vi "test Float Data Integrity.vi"(8 "error in (no error)":errorcluster, 11 "TestCase in":refnum<class "TestCase.lvclass">) -> (0 "error out":errorcluster, 3 "TestCase out":refnum<class "TestCase.lvclass">)   [LabVIEW 2017, in "Pointer Tests.lvlib" / "Data Manipulation Tests.lvclass"]
uses:
  Data Manipulation Tests.lvclass
  <vilib>/addons/_JKI Toolkits/VI Tester/TestCase.llb/TestCase.lvclass
  Source/Classes/Pointer/Write 1D SGL.vi
  Source/Classes/Pointer/Write 1D DBL.vi
  Source/Classes/Pointer/Write SGL.vi
  Source/Classes/Pointer/Write DBL.vi
  Source/Classes/Pointer/Pointer.lvclass
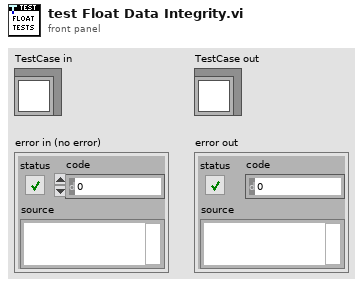
[diagram p1: front panel]
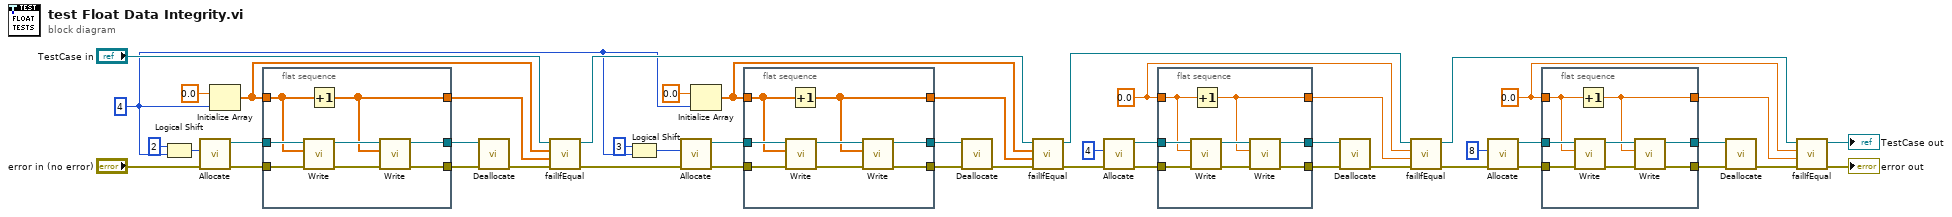
[diagram p0: block diagram]
diagram:
  w5 = u64 4 ("count (1)")
  w22 = 0.0 ("value")
  w11 = sgl 0.0 ("value")
  n1 = Logical Shift(y=i16 2, x=w5) -> (x << y=w8:u64)
  n2 = call "Allocate.vi"("error in (no error)"="error in (no error)", "size"=w8) -> ("error out"=w36:errorcluster, "Pointer out"=w33:refnum<class "Pointer.lvclass">)  [unwired: 8 in]
  n3 = Initialize Array(sgl 0.0 ("element"), w5) -> (w39:sgl[])
  n4 = flat-sequence {
    tunnel: w33 -> [w55]
    tunnel: [w53] -> w34
    tunnel: [w52] -> w35
    tunnel: w36 -> [w50]
    tunnel: w39 -> [w49]
    tunnel: [w48] -> w38
    frame #0 {
      n5 = call-poly "Write.vi"("error in (no error)"=w50, "buffer in"=w49, "Pointer in"=w55) -> ("error out"=w51:errorcluster, "Pointer out"=w54:refnum<class "Pointer.lvclass">)  [unwired: 5 in, 2 out]
      n6 = Increment(x=w49) -> (x+1=w48:sgl[])
      n7 = call-poly "Write.vi"("error in (no error)"=w51, "buffer in"=w48, "Pointer in"=w54) -> ("error out"=w52:errorcluster, "Pointer out"=w53:refnum<class "Pointer.lvclass">)  [unwired: 5 in, 2 out]
    }
  }
  n8 = call "Deallocate.vi"("error in (no error)"=w35, "Pointer in"=w34) -> ("error out"=w37:errorcluster)  [unwired: 8 in, 1 out]
  n9 = call-dynamic "failIfEqual.vi"("error in (no error)"=w37, "y"=w38, "x"=w39, "TestCase in"="TestCase in") -> ("error out"=w26:errorcluster, "TestCase out"=w27:refnum<class "TestCase.lvclass">)  [unwired: 6 in]
  n10 = Logical Shift(y=i16 3, x=w5) -> (x << y=w4:u64)
  n11 = call "Allocate.vi"("error in (no error)"=w26, "size"=w4) -> ("error out"=w29:errorcluster, "Pointer out"=w32:refnum<class "Pointer.lvclass">)  [unwired: 8 in]
  n12 = Initialize Array(0.0 ("value"), w5) -> (w42:dbl[])
  n13 = flat-sequence {
    tunnel: w32 -> [w63]
    tunnel: [w61] -> w31
    tunnel: [w60] -> w30
    tunnel: w29 -> [w58]
    tunnel: w42 -> [w57]
    tunnel: [w56] -> w1
    frame #0 {
      n14 = call-poly "Write.vi"("error in (no error)"=w58, "buffer in"=w57, "Pointer in"=w63) -> ("error out"=w59:errorcluster, "Pointer out"=w62:refnum<class "Pointer.lvclass">)  [unwired: 5 in, 2 out]
      n15 = Increment(x=w57) -> (x+1=w56:dbl[])
      n16 = call-poly "Write.vi"("error in (no error)"=w59, "buffer in"=w56, "Pointer in"=w62) -> ("error out"=w60:errorcluster, "Pointer out"=w61:refnum<class "Pointer.lvclass">)  [unwired: 5 in, 2 out]
    }
  }
  n17 = call "Deallocate.vi"("error in (no error)"=w30, "Pointer in"=w31) -> ("error out"=w28:errorcluster)  [unwired: 8 in, 1 out]
  n18 = call-dynamic "failIfEqual.vi"("error in (no error)"=w28, "y"=w1, "x"=w42, "TestCase in"=w27) -> ("error out"=w44:errorcluster, "TestCase out"=w47:refnum<class "TestCase.lvclass">)  [unwired: 6 in]
  n19 = call "Allocate.vi"("error in (no error)"=w44, "size"=u64 4) -> ("error out"=w13:errorcluster, "Pointer out"=w16:refnum<class "Pointer.lvclass">)  [unwired: 8 in]
  n20 = flat-sequence {
    tunnel: w16 -> [w71]
    tunnel: [w69] -> w15
    tunnel: [w68] -> w14
    tunnel: w13 -> [w66]
    tunnel: w11 -> [w65]
    tunnel: [w64] -> w10
    frame #0 {
      n21 = call-poly "Write.vi"("error in (no error)"=w66, "value"=w65, "Pointer in"=w71) -> ("error out"=w67:errorcluster, "Pointer out"=w70:refnum<class "Pointer.lvclass">)  [unwired: 5 in, 2 out]
      n22 = Increment(x=w65) -> (x+1=w64:sgl)
      n23 = call-poly "Write.vi"("error in (no error)"=w67, "value"=w64, "Pointer in"=w70) -> ("error out"=w68:errorcluster, "Pointer out"=w69:refnum<class "Pointer.lvclass">)  [unwired: 5 in, 2 out]
    }
  }
  n24 = call "Deallocate.vi"("error in (no error)"=w14, "Pointer in"=w15) -> ("error out"=w12:errorcluster)  [unwired: 8 in, 1 out]
  n25 = call-dynamic "failIfEqual.vi"("error in (no error)"=w12, "y"=w10, "x"=w11, "TestCase in"=w47) -> ("error out"=w25:errorcluster, "TestCase out"=w24:refnum<class "TestCase.lvclass">)  [unwired: 6 in]
  n26 = call "Allocate.vi"("error in (no error)"=w25, "size"=u64 8) -> ("error out"=w20:errorcluster, "Pointer out"=w17:refnum<class "Pointer.lvclass">)  [unwired: 8 in]
  n27 = flat-sequence {
    tunnel: w17 -> [w79]
    tunnel: [w77] -> w18
    tunnel: [w76] -> w19
    tunnel: w20 -> [w74]
    tunnel: w22 -> [w73]
    tunnel: [w72] -> w23
    frame #0 {
      n28 = call-poly "Write.vi"("error in (no error)"=w74, "value"=w73, "Pointer in"=w79) -> ("error out"=w75:errorcluster, "Pointer out"=w78:refnum<class "Pointer.lvclass">)  [unwired: 5 in, 2 out]
      n29 = Increment(x=w73) -> (x+1=w72:dbl)
      n30 = call-poly "Write.vi"("error in (no error)"=w75, "value"=w72, "Pointer in"=w78) -> ("error out"=w76:errorcluster, "Pointer out"=w77:refnum<class "Pointer.lvclass">)  [unwired: 5 in, 2 out]
    }
  }
  n31 = call "Deallocate.vi"("error in (no error)"=w19, "Pointer in"=w18) -> ("error out"=w21:errorcluster)  [unwired: 8 in, 1 out]
  n32 = call-dynamic "failIfEqual.vi"("error in (no error)"=w21, "y"=w23, "x"=w22, "TestCase in"=w24) -> ("error out"=→"error out":errorcluster, "TestCase out"=→"TestCase out":refnum<class "TestCase.lvclass">)  [unwired: 6 in]
